vi "Rake Line Profile.vi"() -> ()   [LabVIEW 2024]
doc: "An example on creating rake line profiles, edge detection and line fit in images.\nThis is done in several steps in order for developers to implement custom deviations on the profile, edge detection and line fit algorithms."
uses:
  <vilib>/Natan Biesmans/G2CPU GPU and CPU HPC Toolkit/G2CPU Libraries/File IO/G2CPU File IO.lvlib
  39236cb1-4421-4632-9793-879c1fad6800.vi
  G2CPU Line Profile.lvlib
  5a47bb14-2d54-442f-b15e-951d99135e2c.vi
  8a365540-2057-4560-b5fa-0d389d25a5b7.vi
  a8b570a5-0018-4766-b685-dd53d51ee801.vi
  75f308b9-23f4-4599-bb70-b05a4ad78037.vi
  ce1ec001-2c7f-4b3b-bb82-b025622a0ab9.vi
  c1761f8d-2f54-4d00-9b5e-a0891ec4f845.vi
  d87f0f04-805f-4397-ab8b-1060b47bd9e6.vi
  51ee4c82-ffad-4a24-9029-be6fb9ccb585.vi
  <vilib>/Natan Biesmans/G2CPU GPU and CPU HPC Toolkit/G2CPU Libraries/Arrays/1DArray/s32/1D Array s32.lvclass
  <vilib>/Natan Biesmans/G2CPU GPU and CPU HPC Toolkit/G2CPU Libraries/Arrays/1DArray/f32/1D Array f32.lvclass
  ea995310-c441-49ab-890f-857dd100179f.vi
  723accd1-4565-47a6-94e3-acaea7e77a5d.vi
  4cf4df1d-d6d9-4dcc-8bf6-daa5f74721e9.vi
  3b8c853d-7a23-47f8-bb4a-1c136ef0f793.vi
  7f8f2bde-398a-4b3a-b36e-d4e8a06aa3be.vi
  ffdd45fb-dd29-4cfd-981c-754966d51900.vi
  f53f8924-df60-4935-9a11-a690c02458ae.vi
  858be02d-e4b3-40f0-92f9-edac9443e6ea.vi
  825682f7-b07b-407b-a5ef-2d970f19d533.vi
  d7da47b7-008d-4b91-9fb2-11c2935ac586.vi
  1de05a6f-66a6-4443-9878-c56794eee180.vi
  8da2aec0-933a-4f35-b4cb-24f00b3d5aa1.vi
  <vilib>/Natan Biesmans/G2CPU GPU and CPU HPC Toolkit/G2CPU Libraries/Arrays/1DArray/binary/1D Array binary.lvclass
  <vilib>/Natan Biesmans/G2CPU GPU and CPU HPC Toolkit/G2CPU Libraries/File IO/Images/G2CPU Load 32b Image.vi
panel:
  in  "Px 3":sgl[](array[numeric])=[290.0, 20.0] format="%#_g px"
  in  "Py 3":sgl[](array[numeric])=[310.0, 140.0] format="%#_g px"
  in  "Rising Edge":bool[](array[boolean])=[TRUE, FALSE]
  in  "Amounts of Lines":i32[](array[numeric])=[20, 20]
  in  "Treshold":i32[](array[numeric])=[50, 50]
  in  "Py 2":sgl[](array[numeric])=[300.0, 130.0] format="%#_g px"
  in  "Px 2":sgl[](array[numeric])=[470.0, 230.0] format="%#_g px"
  in  "Py 1":sgl[](array[numeric])=[210.0, 30.0] format="%#_g px"
  in  "Px 1":sgl[](array[numeric])=[340.0, 100.0] format="%#_g px"
  in  "Image File":path=path "C:/Program Files/ArrayFire/v3/examples/images/atlantis.png"
  out "Fit Keys":u32[](array[numeric])
  out "C":sgl[](array[numeric]) format="%.2f"
  out "B":sgl[](array[numeric]) format="%.2f"
  out "A":sgl[](array[numeric]) format="%.2f"
  out "Original Image":sgl[][](graph)
  out "Line Profiles":sgl[][](graph)
  # "Rake Position"
  # "Edge Detection Parameters"
  # "Line fit on rake"
  # "A * x + B * y + C = 0"
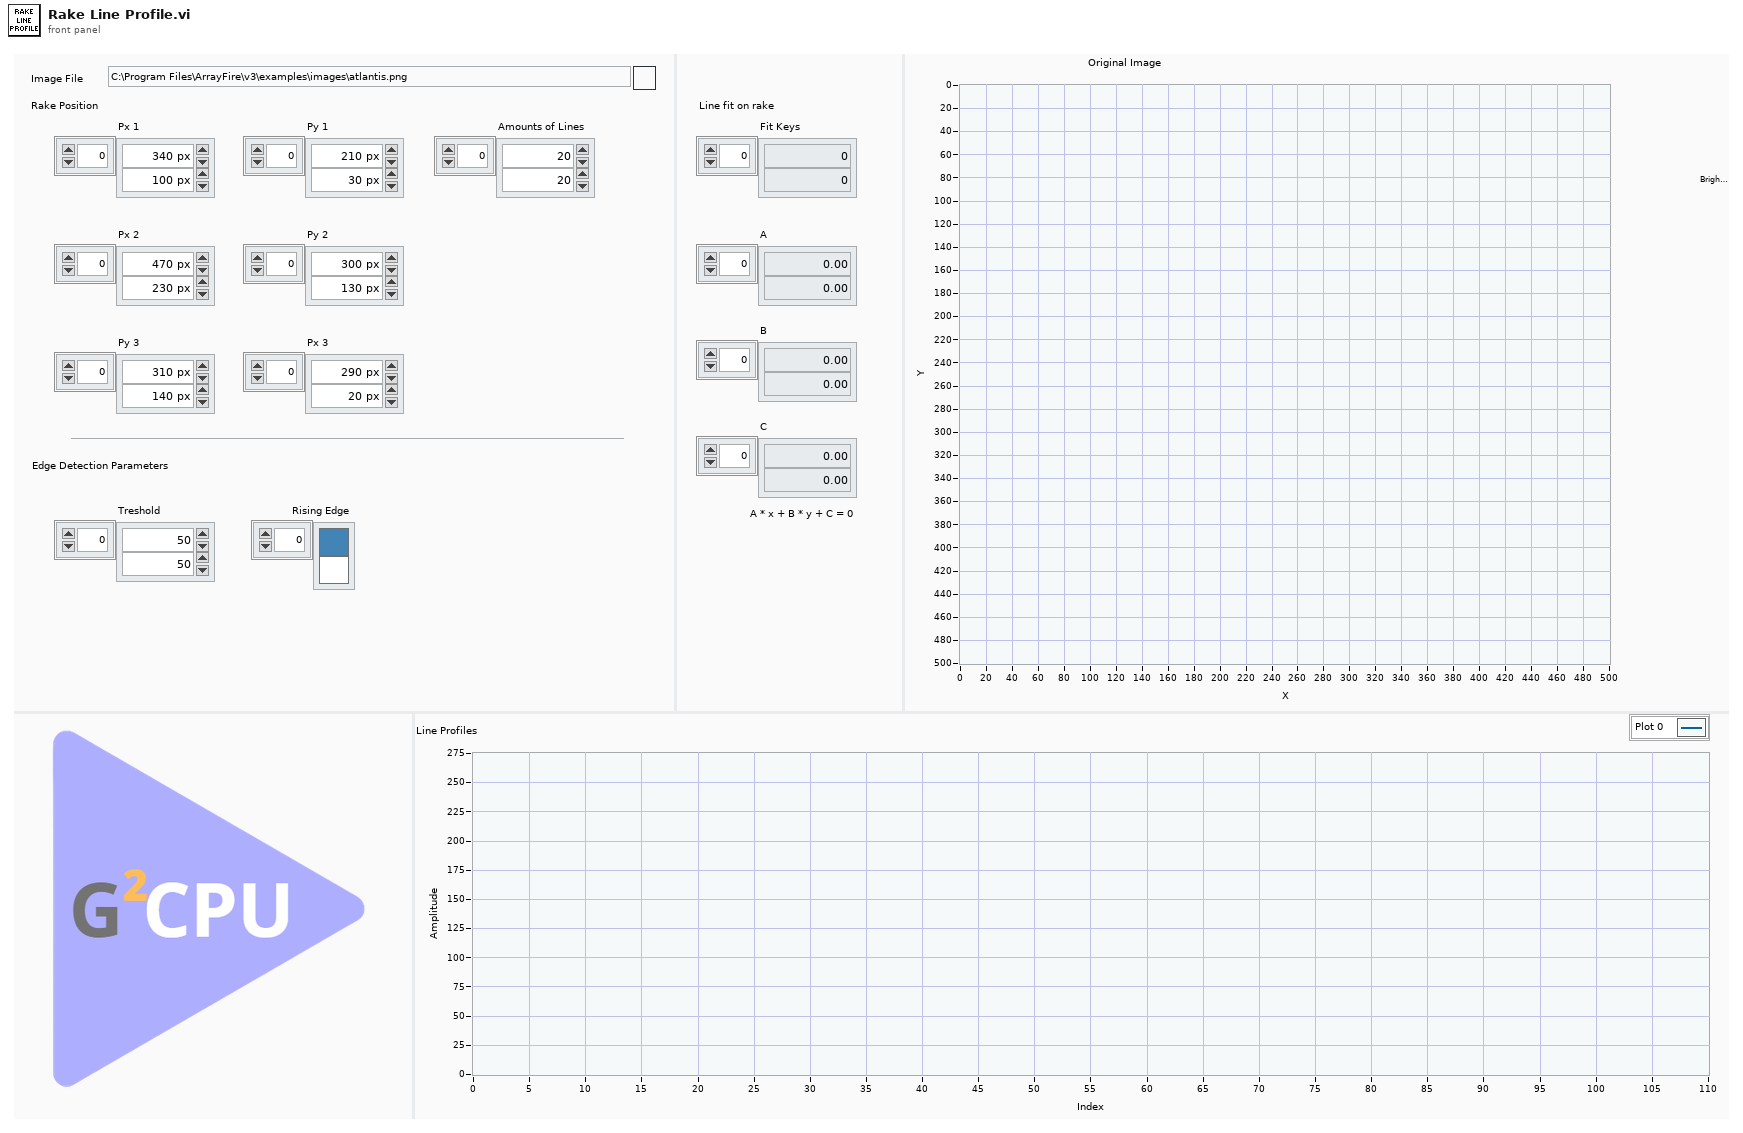
[diagram p1: front panel]
types:
  T1 = cluster{"Auto Release Line Indexers (Enabled)":bool, "Auto Release Keys (Enabled)":bool}
  T2 = cluster{"Rising Edge?":refnum<class "1D Array binary.lvclass">, "Treshold":refnum<class "1D Array s32.lvclass">}
  T3 = cluster{"Px 1":refnum<class "1D Array f32.lvclass">, "Py 1":refnum<class "1D Array f32.lvclass">, "Px 2":refnum<class "1D Array f32.lvclass">, "Py 2":refnum<class "1D Array f32.lvclass">, "Px 3":refnum<class "1D Array f32.lvclass">, "Py 3":refnum<class "1D Array f32.lvclass">, "Amount of Lines":refnum<class "1D Array s32.lvclass">}
  T4 = cluster{"Points 1 X":refnum<class "1D Array f32.lvclass">, "Points 1 Y":refnum<class "1D Array f32.lvclass">, "Points 2 X":refnum<class "1D Array f32.lvclass">, "Points 2 Y":refnum<class "1D Array f32.lvclass">, "Keys":refnum<class "1D Array u32.lvclass">}
  T5 = cluster{"Line Indexes":refnum<class "2D Array f32.lvclass">, "Keys":refnum<class "2D Array u32.lvclass">, "Index Overflow":u64}
  T6 = cluster{"Line Profiles":refnum<class "2D Array f32.lvclass">, "Keys":refnum<class "2D Array u32.lvclass">}
  T7 = cluster{"X Coordinates":refnum<class "1D Array f32.lvclass">, "Y Coordinates":refnum<class "1D Array f32.lvclass">, "Keys":refnum<class "1D Array u32.lvclass">}
  T8 = cluster{"A(x)":refnum<class "1D Array f32.lvclass">, "B(y)":refnum<class "1D Array f32.lvclass">, "C":refnum<class "1D Array f32.lvclass">, "Keys Out":refnum<class "1D Array u32.lvclass">}
  T9 = cluster{"Name":string, "Color":u32, "Style":u8, "Point Style":u8, "Name Visible":bool, "Allow Drag":bool, "Annotation Mode":u32, "Plot":i32, "Index":i32, "Position":cluster{"X":dbl, "Y":dbl}, "X Scale":u32, "Y Scale":u32, "Show Arrow":bool, "Lock Name":bool, "Plot Area":i32, "Label Offset":cluster{"X":dbl, "Y":dbl}}
  T10 = cluster{"Name":string, "Color":u32, "Style":u8, "Point Style":u8, "Name Visible":bool, "Allow Drag":bool, "Annotation Mode":u32, "Plot":i32, "Index":i32, "Position":cluster{"X":dbl, "Y":dbl}, "X Scale":u32, "Y Scale":u32, "Show Arrow":bool, "Lock Name":bool, "Plot Area":i32, "Label Offset":cluster{"X":dbl, "Y":dbl}}[]
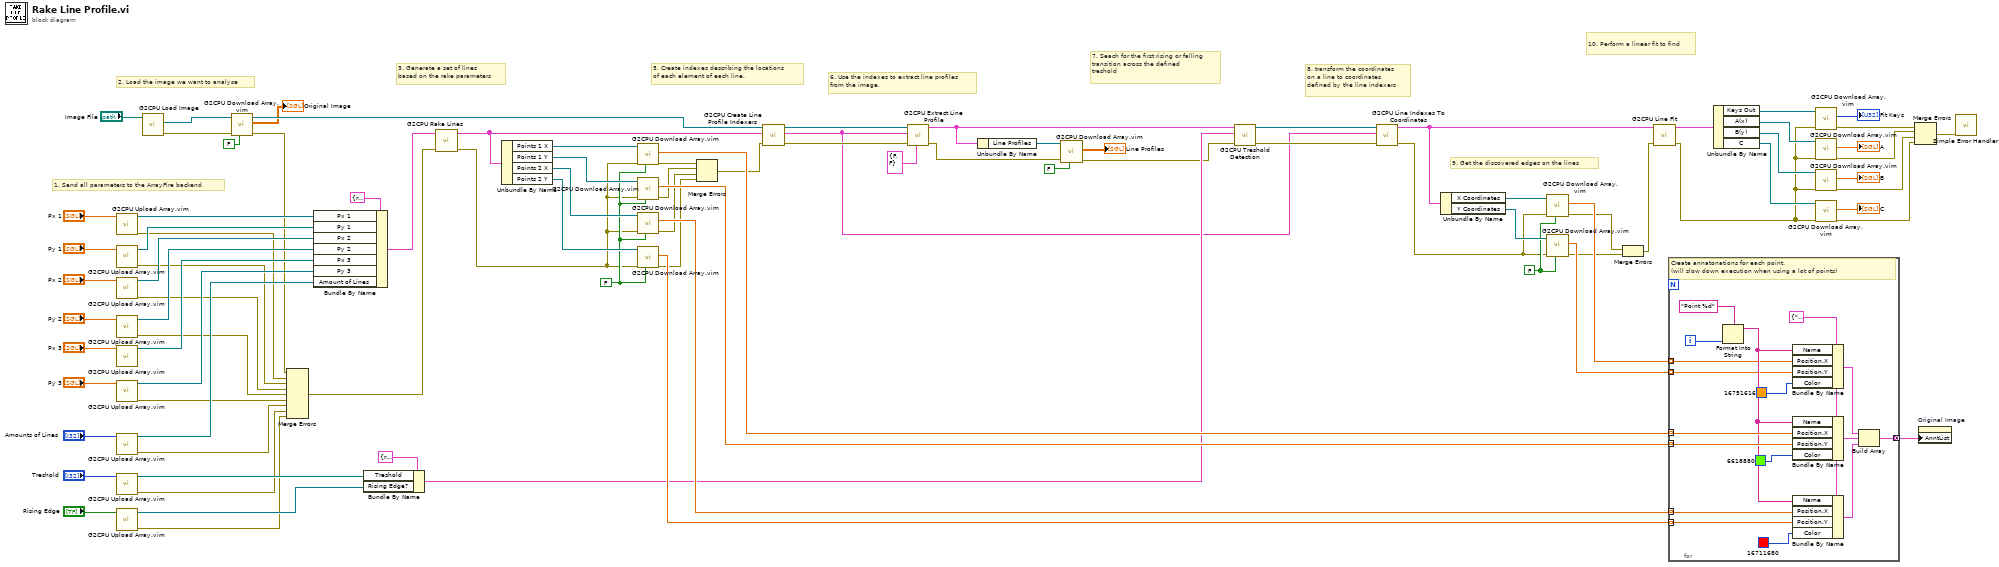
[diagram p0: block diagram]
diagram:
  w51 = FALSE ("Auto Release Array In")
  w79 = FALSE ("Auto Release Array In")
  # "10. Perform a linear fit to find"
  # "9. Get the discovered edges on the lines"
  # "8. transform the coordinates\non a line to coordinates\ndefined by the line indexers"
  # "7. Seach for the first rising or falling\ntransition across the defined \ntreshold"
  # "6. Use the indexes to extract line profiles \nfrom the image."
  # "5. Create indexes describing the locations\nof each element of each line."
  # "3. Generate a set of lines \nbased on the rake parameters"
  # "2. Load the image we want to analyse"
  # "1. Send all parameters to the ArrayFire backend"
  n1 = call "G2CPU Upload Array.vim"("Data"="Px 1") -> ("error out"=w41:errorcluster, "Array"=w72:refnum<class "1D Array f32.lvclass">)  [unwired: 9 in]
  n2 = call "G2CPU Upload Array.vim"("Data"="Py 1") -> ("error out"=w40:errorcluster, "Array"=w71:refnum<class "1D Array f32.lvclass">)  [unwired: 9 in]
  n3 = call "G2CPU Upload Array.vim"("Data"="Px 2") -> ("error out"=w39:errorcluster, "Array"=w70:refnum<class "1D Array f32.lvclass">)  [unwired: 9 in]
  n4 = call "G2CPU Upload Array.vim"("Data"="Py 2") -> ("error out"=w38:errorcluster, "Array"=w69:refnum<class "1D Array f32.lvclass">)  [unwired: 9 in]
  n5 = call "G2CPU Upload Array.vim"("Data"="Px 3") -> ("Array"=w68:refnum<class "1D Array f32.lvclass">)  [unwired: 9 in, 1 out]
  n6 = call "G2CPU Upload Array.vim"("Data"="Py 3") -> ("error out"=w36:errorcluster, "Array"=w67:refnum<class "1D Array f32.lvclass">)  [unwired: 9 in]
  n7 = call "G2CPU Upload Array.vim"("Data"="Amounts of Lines") -> ("error out"=w37:errorcluster, "Array"=w66:refnum<class "1D Array s32.lvclass">)  [unwired: 9 in]
  n8 = call "G2CPU Upload Array.vim"("Data"="Treshold") -> ("error out"=w35:errorcluster, "Array"=w56:refnum<class "1D Array s32.lvclass">)  [unwired: 9 in]
  n9 = call "G2CPU Upload Array.vim"("Data"="Rising Edge") -> ("error out"=w34:errorcluster, "Array"=w55:refnum<class "1D Array binary.lvclass">)  [unwired: 9 in]
  n10 = call-poly <vilib>:"G2CPU Load Image.vi"("Filename"="Image File") -> ("error out"=w91:errorcluster, "Array out"=w92:refnum<class "2D Array f32.lvclass">)  [unwired: 7 in, 2 out]
  n11 = call "G2CPU Download Array.vim"("Auto Release Array In"=FALSE, "error in (no error)"=w91, "Array in"=w92) -> ("error out"=w43:errorcluster, "Array Data"=→"Original Image":sgl[][], "Array Out"=w89:refnum<class "2D Array f32.lvclass">)  [unwired: 6 in]
  n12 = Merge Errors(w43, w41, w40, w39, w38, w36, w37, w35, w34) -> (w42:errorcluster)
  n13 = Bundle By Name(cluster=T3 {"Px 1"=refnum, "Py 1"=refnum, "Px 2"=refnum, "Py 2"=refnum, "Px 3"=refnum, "Py 3"=refnum, "Amount of Lines"=refnum} ("Rake Parameters"), "Px 1"=w72, "Py 1"=w71, "Px 2"=w70, "Py 2"=w69, "Px 3"=w68, "Py 3"=w67, "Amount of Lines"=w66) -> (w73:T3)
  n14 = Bundle By Name(cluster=T2 {"Rising Edge?"=refnum, "Treshold"=refnum} ("Treshold Parameters"), "Treshold"=w56, "Rising Edge?"=w55) -> (w49:T2)
  n15 = call "G2CPU Rake Lines.vi"("error in (no error)"=w42, "Rake Parameters"=w73) -> ("error out"=w29:errorcluster, "Lines"=w84:T4)  [unwired: 8 in]
  n16 = Unbundle By Name(w84) -> ("Points 1 X"=w82:refnum<class "1D Array f32.lvclass">, "Points 1 Y"=w81:refnum<class "1D Array f32.lvclass">, "Points 2 X"=w80:refnum<class "1D Array f32.lvclass">, "Points 2 Y"=w83:refnum<class "1D Array f32.lvclass">)
  n17 = call "G2CPU Download Array.vim"("Auto Release Array In"=w79, "error in (no error)"=w29, "Array in"=w82) -> ("error out"=w33:errorcluster, "Array Data"=w75:sgl[])  [unwired: 6 in, 1 out]
  n18 = call "G2CPU Download Array.vim"("Auto Release Array In"=w79, "error in (no error)"=w29, "Array in"=w81) -> ("error out"=w32:errorcluster, "Array Data"=w77:sgl[])  [unwired: 6 in, 1 out]
  n19 = call "G2CPU Download Array.vim"("Auto Release Array In"=w79, "error in (no error)"=w29, "Array in"=w80) -> ("error out"=w31:errorcluster, "Array Data"=w76:sgl[])  [unwired: 6 in, 1 out]
  n20 = call "G2CPU Download Array.vim"("Auto Release Array In"=w79, "error in (no error)"=w29, "Array in"=w83) -> ("error out"=w30:errorcluster, "Array Data"=w78:sgl[])  [unwired: 6 in, 1 out]
  n21 = Merge Errors(w33, w32, w31, w30) -> (w28:errorcluster)
  n22 = call "G2CPU Create Line Profile Indexers.vi"("error in (no error)"=w28, "Lines"=w84, "Greyscale Image In"=w89) -> ("error out"=w48:errorcluster, "Line Indexers"=w45:T5, "Greyscale Image Out (inplace)"=w88:refnum<class "2D Array f32.lvclass">)  [unwired: 6 in]
  n23 = call "G2CPU Extract Line Profile.vi"("Auto Release Line Indexers"=T1 {"Auto Release Line Indexers (Enabled)"=FALSE, "Auto Release Keys (Enabled)"=FALSE}, "error in (no error)"=w48, "Line Indexers"=w45, "Greyscale Image In"=w88) -> ("error out"=w17:errorcluster, "Line Profiles Out"=w65:T6)  [unwired: 6 in]
  n24 = Unbundle By Name(w65) -> ("Line Profiles"=w87:refnum<class "2D Array f32.lvclass">)
  n25 = call "G2CPU Download Array.vim"("Auto Release Array In"=FALSE, "error in (no error)"=w17, "Array in"=w87) -> ("error out"=w16:errorcluster, "Array Data"=→"Line Profiles":sgl[][])  [unwired: 6 in, 1 out]
  n26 = call "G2CPU Treshold Detection.vi"("error in (no error)"=w16, "Treshold Parameters"=w49, "Line Profiles"=w65) -> ("error out"=w47:errorcluster, "Edge Indexes out"=w52:refnum<class "1D Array f32.lvclass">)  [unwired: 7 in]
  n27 = call "G2CPU Line Indexes To Coordinates.vi"("error in (no error)"=w47, "Line Indexers"=w45, "Point of Interest on Lines"=w52) -> ("error out"=w27:errorcluster, "Coordinates Out"=w62:T7)  [unwired: 7 in]
  n28 = Unbundle By Name(w62) -> ("X Coordinates"=w54:refnum<class "1D Array f32.lvclass">, "Y Coordinates"=w53:refnum<class "1D Array f32.lvclass">)
  n29 = call "G2CPU Download Array.vim"("Auto Release Array In"=w51, "error in (no error)"=w27, "Array in"=w54) -> ("error out"=w25:errorcluster, "Array Data"=w86:sgl[])  [unwired: 6 in, 1 out]
  n30 = call "G2CPU Download Array.vim"("Auto Release Array In"=w51, "error in (no error)"=w27, "Array in"=w53) -> ("error out"=w26:errorcluster, "Array Data"=w85:sgl[])  [unwired: 6 in, 1 out]
  n31 = Merge Errors(w25, w26) -> (w24:errorcluster)
  n32 = call "G2CPU Line Fit.vi"("error in"=w24, "Coordinates In"=w62) -> ("error out"=w23:errorcluster, "Fits Out"=w61:T8)  [unwired: 8 in]
  n33 = for {
    tunnel: [w105] -> w63 mode=concatenating
    tunnel: w75 -> [w102] mode=indexing
    tunnel: w77 -> [w101] mode=indexing
    tunnel: w76 -> [w100] mode=indexing
    tunnel: w78 -> [w99] mode=indexing
    tunnel: w86 -> [w95] mode=indexing
    tunnel: w85 -> [w94] mode=indexing
    i -> [w104]
    w97 = T9 {"Name"="azerty", "Color"=16776960, "Style"=4, "Point Style"=13, "Name Visible"=FALSE, "Allow Drag"=TRUE, "Annotation Mode"=0, "Plot"=-1, "Index"=0, "Position"={"X"=162.8968713789108, "Y"=222.19554030874787}, "X Scale"=0, "Y Scale"=0, "Show Arrow"=TRUE, "Lock Name"=FALSE, "Plot Area"=0, "Label Offset"={"X"=0.0, "Y"=-11.663807890222984}}
    # "Create annatonations for each point.\n(will slow down execution when using a lot of points)"
    n34 = Format Into String(format string="Point %d", w104) -> (resulting string=w96:string)  [unwired: 2 in, 1 out]
    n35 = Bundle By Name(cluster=w97, "Name"=w96, "Position.X"=w95, "Position.Y"=w94, "Color"=u32 16751616) -> (w93:T9)
    n36 = Bundle By Name(cluster=w97, "Name"=w96, "Position.X"=w102, "Position.Y"=w101, "Color"=u32 6618880) -> (w106:T9)
    n37 = Bundle By Name(cluster=w97, "Name"=w96, "Position.X"=w100, "Position.Y"=w99, "Color"=u32 16711680) -> (w107:T9)
    n38 = Build Array(w93, w106, w107) -> (w105:T10)
  }
  n39 = Unbundle By Name(w61) -> ("Keys Out"=w60:refnum<class "1D Array u32.lvclass">, "A(x)"=w59:refnum<class "1D Array f32.lvclass">, "B(y)"=w58:refnum<class "1D Array f32.lvclass">, "C"=w57:refnum<class "1D Array f32.lvclass">)
  n40 = call "G2CPU Download Array.vim"("error in (no error)"=w23, "Array in"=w60) -> ("error out"=w22:errorcluster, "Array Data"=→"Fit Keys":u32[])  [unwired: 7 in, 1 out]
  n41 = call "G2CPU Download Array.vim"("error in (no error)"=w23, "Array in"=w59) -> ("error out"=w21:errorcluster, "Array Data"=→"A":sgl[])  [unwired: 7 in, 1 out]
  n42 = call "G2CPU Download Array.vim"("error in (no error)"=w23, "Array in"=w58) -> ("error out"=w20:errorcluster, "Array Data"=→"B":sgl[])  [unwired: 7 in, 1 out]
  n43 = call "G2CPU Download Array.vim"("error in (no error)"=w23, "Array in"=w57) -> ("error out"=w19:errorcluster, "Array Data"=→"C":sgl[])  [unwired: 7 in, 1 out]
  n44 = Merge Errors(w22, w21, w20, w19) -> (w14:errorcluster)
  n45 = property on="Original Image" class="IntGraph (strict)"("AnntList"=w63) -> ()  [unwired: 2 in, 2 out]
  n46 = call <vilib>:"Simple Error Handler.vi"("error in (no error)"=w14) -> ()  [unwired: 4 in, 5 out]
